vi "MicroStrain 3DM-GXx Calibration.vi"() -> ()   [LabVIEW 2012]
doc: "Shows how to setup the device and configure the gyro and accelerometer offsets."
uses:
  <instrlib>/MicroStrain 3DM-GXx/MicroStrain 3DM-GXx.lvlib
panel:
  in  "Z Axis Accelerometer Offset  (0 m/s^2)":sgl
  in  "Y Axis Accelerometer Offset  (0 m/s^2)":sgl
  in  "X Axis Accelerometer Offset (0 m/s^2)":sgl
  in  "Sample Time (10000 ms)":u16=10000
  in  "VISA resource name":refnum<visa-resource-name>
  # "(c) 2009 - 2011 National Instruments.  ALL RIGHTS RESERVED."
  # "This VI demonstrates the process of calibrating the device.  \nThe Gyro offset is automatically calculated and stored in RAM. \nThe Accelerometer offset is entered manually and stored in RAM. \nTo save these values to non-volatile EEPROM use the 'Transfer Calibration To EERPOM' VI."
  # "Enter the accelerometer offset to be written to the device. \nThis offset will be subtracted from all subsequent measurements\nof acceleration.  This value will be stored in RAM but can be \ntransferred to EEPROM using the 'Transfer Calibration To EEPROM' VI."
  # "Enter the amount of time for the device to sample its\nsensors to determine the gyro offset.  Recommended \nsample times are between 10,000 and 30,000 ms.\n*The device must remain stationary during this time."
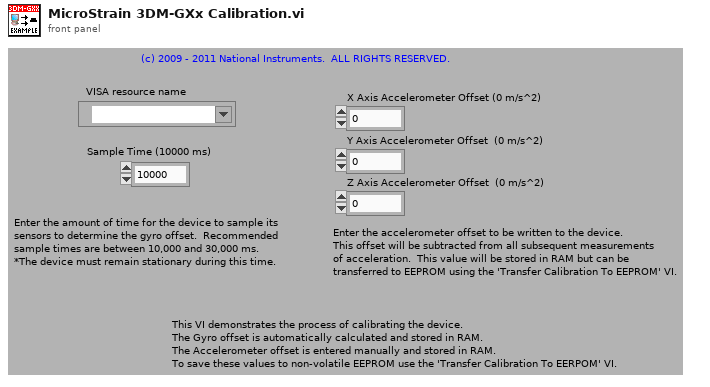
[diagram p1: front panel]
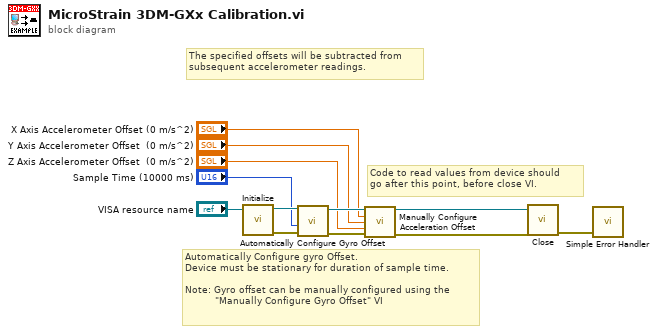
[diagram p0: block diagram]
diagram:
  # "Code to read values from device should \ngo after this point, before close VI."
  # "The specified offsets will be subtracted from\nsubsequent accelerometer readings."
  # "Automatically Configure gyro Offset.\nDevice must be stationary for duration of sample time.\n\nNote: Gyro offset can be manually configured using the\n          \"Manually Configure Gyro Offset\" VI"
  n1 = call <instrlib>:"Initialize.vi"("VISA resource name"="VISA resource name") -> ("error out"=w11:errorcluster, "VISA resource name out"=w12:refnum<visa-resource-name>)  [unwired: 9 in]
  n2 = call <instrlib>:"Automatically Configure Gyro Offset.vi"("error in (no error)"=w11, "Sample Time (10000 ms)"="Sample Time (10000 ms)", "VISA resource name"=w12) -> ("error out"=w5:errorcluster, "VISA resource name out"=w8:refnum<visa-resource-name>)  [unwired: 7 in]
  n3 = call <instrlib>:"Manually Configure Acceleration Offset.vi"("VISA resource name"=w8, "X Axis Accelerometer Offset (0 m/s^2)"="X Axis Accelerometer Offset (0 m/s^2)", "Y Axis Accelerometer Offset  (0 m/s^2)"="Y Axis Accelerometer Offset  (0 m/s^2)", "Z Axis Accelerometer Offset  (0 m/s^2)"="Z Axis Accelerometer Offset  (0 m/s^2)", "error in (no error)"=w5) -> ("VISA resource name out"=w7:refnum<visa-resource-name>, "error out"=w6:errorcluster)  [unwired: 9 in]
  n4 = call <instrlib>:"Close.vi"("error in (no error)"=w6, "VISA resource name"=w7) -> ("error out"=w9:errorcluster)  [unwired: 9 in]
  n5 = call <vilib>:"Simple Error Handler.vi"("error in (no error)"=w9) -> ()  [unwired: 4 in, 5 out]
